vi "Get Mentions Old.vi"(8 "error in":errorcluster, 9 "Mentions to Read (10)":i32=10 min=0 max=200 step=1, 11 "Twitter Handle In":T2={"OAuth Credentials"={"Consumer Key"="", "Signature Method"=enum."HMAC-SHA1", "Token"="", "Version"="", "Token Secret"="", "Consumer Secret"=""}, "since ID"="", "max ID"="", "Screen Name"=""}) -> (0 "error out":errorcluster, 1 "Actual Num of Mentions Read":i32, 2 "Old Mentions Read":T1[](array[typedef]), 3 "Twitter Handle Out":T2={"OAuth Credentials"={"Consumer Key"="", "Signature Method"=enum."HMAC-SHA1", "Token"="", "Version"="", "Token Secret"="", "Consumer Secret"=""}, "since ID"="", "max ID"="", "Screen Name"=""}, 5 "Time Stamp of Oldest Mention":timestamp)   [LabVIEW 2011, in "i3-twitter.lvlib"]
doc: "Get authenticating user's old mentions."
uses:
  i3-twitter.lvlib
  Controls/Twitter Handle.ctl
  i3-oauth/Controls/OAuth Credentials.ctl
  i3-oauth/Controls/Signature Method.ctl
  Controls/Tweet.ctl
  i3-oauth/Controls/HTTP Method.ctl
  i3-oauth/i3-oauth.lvlib
  <vilib>/httpClient/LabVIEWHTTPClient.lvlib
  i3-json/i3-json.lvlib
panel:
  out "headers":string
  out "body":string
  out "Full URL":string
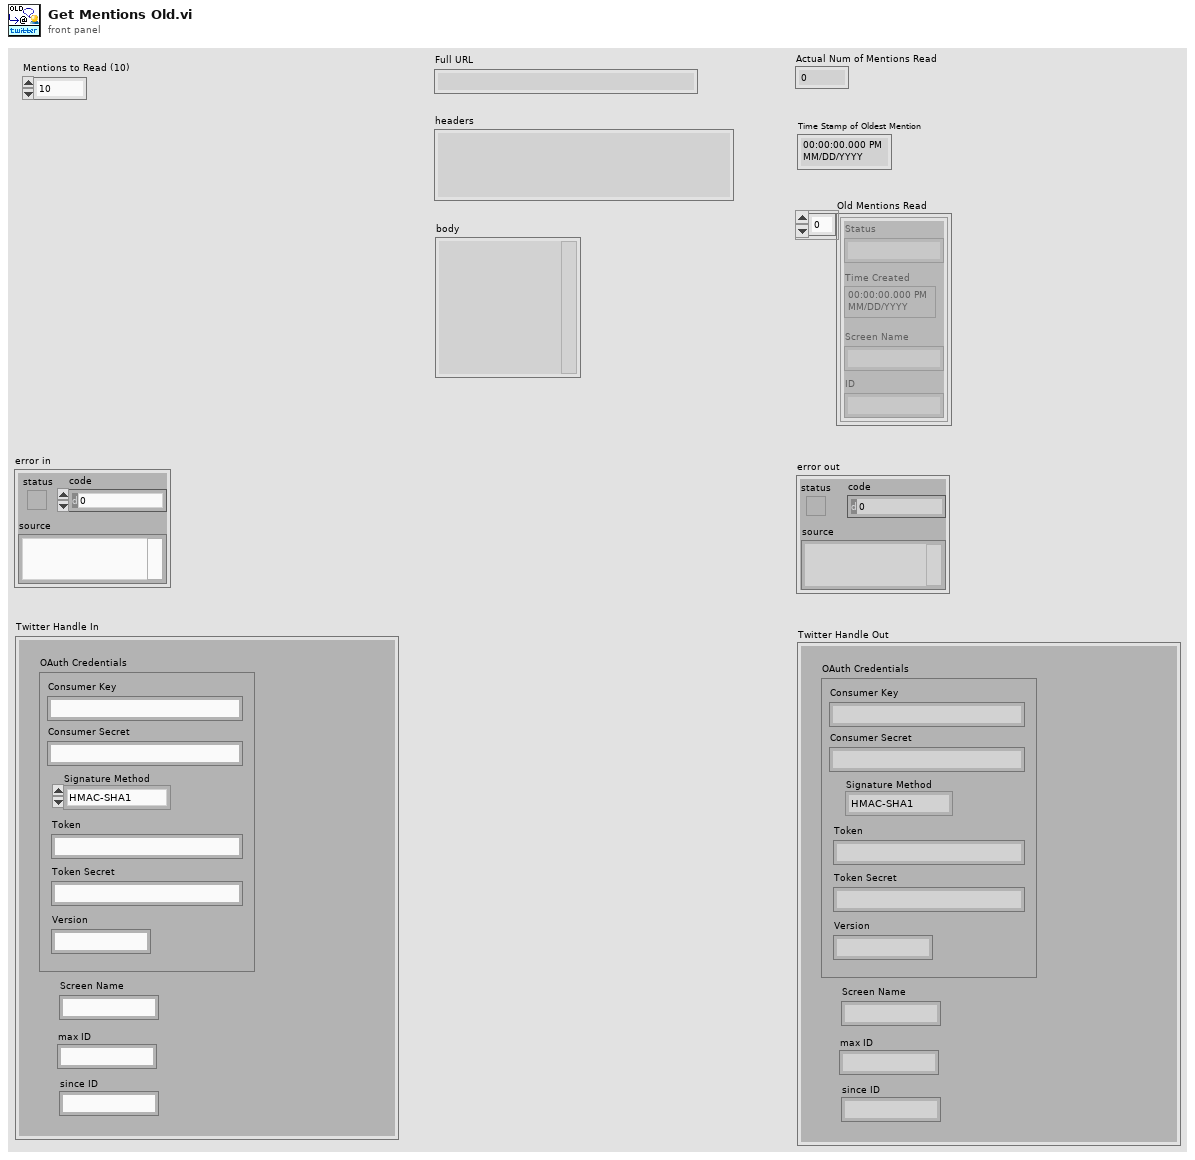
[diagram p1: front panel]
types:
  T1 = typedef "i3-twitter.lvlib/Tweet.ctl" = cluster{"Status":string, "Time Created":timestamp, "Screen Name":string, "ID":string}
  T2 = typedef "i3-twitter.lvlib/Twitter Handle.ctl" = cluster{"OAuth Credentials":T3, "since ID":string, "max ID":string, "Screen Name":string}
  T3 = typedef "i3-oauth.lvlib/OAuth Credentials.ctl" = cluster{"Consumer Key":string, "Signature Method":T4, "Token":string, "Version":string, "Token Secret":string, "Consumer Secret":string}
  T4 = typedef "i3-oauth.lvlib/Signature Method.ctl" = enum16{"HMAC-MD5", "HMAC-SHA1", "HMAC-SHA224", "HMAC-SHA256", "HMAC-SHA384", "HMAC-SHA512"}
  T5 = typedef "i3-oauth.lvlib/HTTP Method.ctl" = enum16{"GET", "POST", "PUT", "DELETE"}
  T6 = typedef "i3-oauth.lvlib/key-value-pairs.ctl" = cluster{"key":string, "value":string}
  T7 = typedef "LabVIEWHTTPClient.lvlib/ClientHandle.ctl" = refnum<k1>
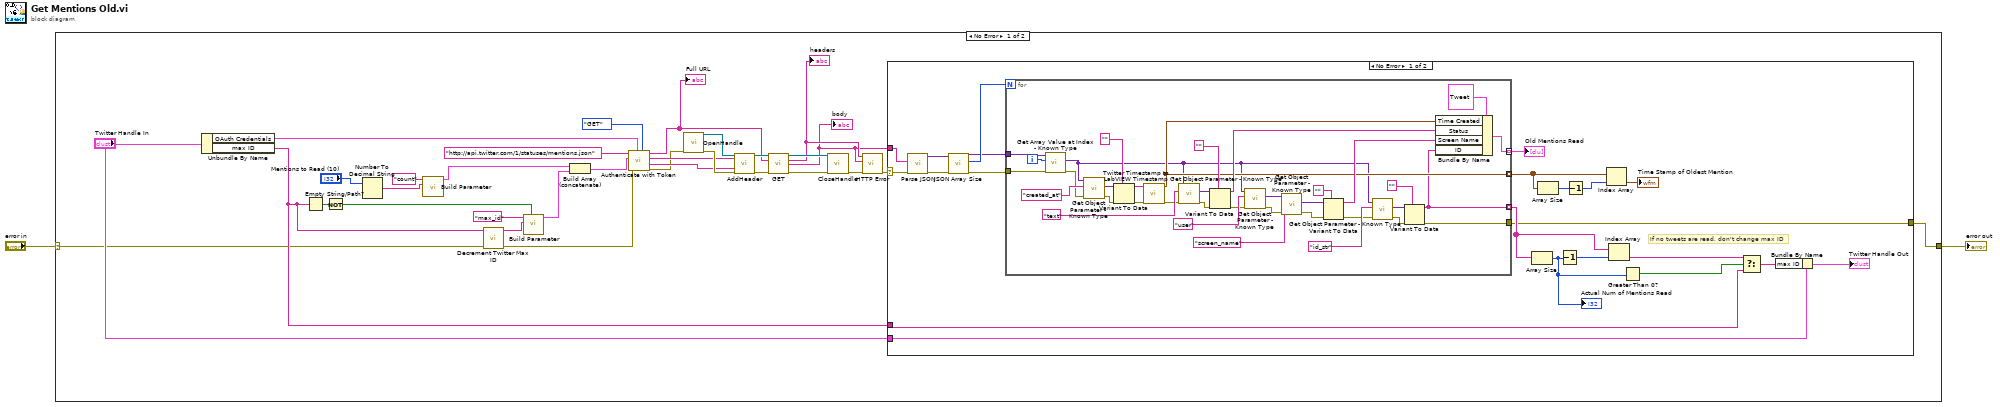
[diagram p0: block diagram]
diagram:
  n1 = case shown="No Error" "error in" {
    selector: "error in" -> [w3 w94]
    tunnel: [w4 w94] -> w2
    frame No Error {
      n2 = Unbundle By Name("Twitter Handle In") -> ("OAuth Credentials"=w8:T3, "max ID"=w6:string)
      n3 = Empty String/Path?(string/path=w6) -> (empty?=w18:bool)
      n4 = Not(x=w18) -> (.not. x?=w14:bool)
      n5 = Number To Decimal String(number="Mentions to Read (10)") -> (decimal integer string=w21:string)  [unwired: 1 in]
      n6 = call "Build Parameter.vi"("Value"=w21, "Key"="count") -> ("Parameter Array"=w7:T6[])  [unwired: 9 in]
      n7 = call "Decrement Twitter Max ID.vi"("error in (no error)"=w3, "ID In"=w6) -> ("error out"=w13:errorcluster, "ID Out"=w15:string)  [unwired: 8 in]
      n8 = call "Build Parameter.vi"("Return Parameter? (T)"=w14, "Value"=w15, "Key"="max_id") -> ("Parameter Array"=w17:T6[])  [unwired: 8 in]
      n9 = Build Array (concatenate)(w7, w17) -> (w20:T6[])
      n10 = call "Authenticate with Token.vi"("HTTP Method"=HTTP_Method."GET", "OAuth Credentials"=w8, "error in (no error)"=w13, "URL Parameters"=w20, "Base URL"="http://api.twitter.com/1/statuses/mentions.json") -> ("error out"=w19:errorcluster, "Header Value"=w26:string, "Header Parameter"=w27:string, "Full URL"=w24:string)  [unwired: 2 in, 1 out]
      "Full URL" <- w24
      n11 = call <vilib>:"OpenHandle.vi"("error in (no error)"=w19) -> ("client handle out"=w33:T7, "error out"=w32:errorcluster)  [unwired: 13 in]
      n12 = call <vilib>:"AddHeader.vi"("client handle"=w33, "header"=w27, "value"=w26, "error in (no error)"=w32) -> ("client handle out"=w31:T7, "error out"=w30:errorcluster)  [unwired: 10 in]
      n13 = call <vilib>:"GET.vi"("client handle"=w31, "url"=w24, "error in (no error)"=w30) -> ("client handle out"=w29:T7, "headers"=w12:string, "body"=w9:string, "error out"=w28:errorcluster)  [unwired: 9 in]
      "body" <- w9
      "headers" <- w12
      n14 = call <vilib>:"CloseHandle.vi"("client handle"=w29, "error in (no error)"=w28) -> ("error out"=w11:errorcluster)  [unwired: 13 in]
      n15 = call "HTTP Error.vi"("error in (no error)"=w11, "Body"=w9, "Header"=w12) -> ("error out"=w10:errorcluster)  [unwired: 6 in, 2 out]
      n16 = case shown="No Error" w10 {
        selector: w10 -> [w42 w93]
        tunnel: w6 -> [w45 _]
        tunnel: "Twitter Handle In" -> [w44 _]
        tunnel: [w39 w93] -> w4
        tunnel: w9 -> [w41 _]
        frame No Error {
          # "If no tweets are read, don't change max ID"
          n17 = call "Parse JSON.vi"("error in (no error)"=w42, "JSON String"=w41) -> ("error out"=w53:errorcluster, "JSON Tree"=w55:variant)  [unwired: 6 in, 2 out]
          n18 = call "JSON Array Size.vi"("error in (no error)"=w53, "JSON Tree In (JSON Array)"=w55) -> ("error out"=w52:errorcluster, "Array Size"=w56:i32, "JSON Tree Passthrough (JSON Array)"=w46:variant)  [unwired: 7 in]
          n19 = for {
            N: w56 -> [_]
            tunnel: [w59] -> w54 mode=indexing
            tunnel: w52 -> [w62]
            tunnel: [w72] -> w51 mode=indexing
            tunnel: [w71] -> w39
            tunnel: w46 -> [w61]
            tunnel: [w60] -> w37 mode=indexing
            i -> [w81]
            n20 = call "Get Array Value at Index - Known Type.vi"("error in (no error)"=w62, "Index"=w81, "JSON Tree In (JSON Array)"=w61) -> ("error out"=w75:errorcluster, "Value"=w58:variant)  [unwired: 3 in, 4 out]
            n21 = call "Get Object Parameter - Known Type.vi"("error in (no error)"=w75, "Parameter Name"="created_at", "JSON Tree In (JSON Object)"=w58) -> ("error out"=w70:errorcluster, "Value"=w68:variant)  [unwired: 3 in, 4 out]
            n22 = Variant To Data(error in=w70, type="", Variant=w68) -> (data=w80:string, error out=w66:errorcluster)
            n23 = call "Twitter Timestamp to LabVIEW Timestamp.vi"("error in"=w66, "Twitter Time Stamp"=w80) -> ("error out"=w65:errorcluster, "LabVIEW Time Stamp"=w60:timestamp)  [unwired: 6 in]
            n24 = call "Get Object Parameter - Known Type.vi"("error in (no error)"=w65, "Parameter Name"="text", "JSON Tree In (JSON Object)"=w58) -> ("error out"=w69:errorcluster, "Value"=w90:variant)  [unwired: 3 in, 4 out]
            n25 = Variant To Data(error in=w69, type="", Variant=w90) -> (data=w63:string, error out=w67:errorcluster)
            n26 = call "Get Object Parameter - Known Type.vi"("error in (no error)"=w67, "Parameter Name"="user", "JSON Tree In (JSON Object)"=w58) -> ("error out"=w74:errorcluster, "Value"=w57:variant)  [unwired: 3 in, 4 out]
            n27 = call "Get Object Parameter - Known Type.vi"("error in (no error)"=w74, "Parameter Name"="screen_name", "JSON Tree In (JSON Object)"=w57) -> ("error out"=w73:errorcluster, "Value"=w85:variant)  [unwired: 3 in, 4 out]
            n28 = Variant To Data(error in=w73, type="", Variant=w85) -> (data=w86:string, error out=w64:errorcluster)
            n29 = call "Get Object Parameter - Known Type.vi"("error in (no error)"=w64, "Parameter Name"="id_str", "JSON Tree In (JSON Object)"=w58) -> ("error out"=w78:errorcluster, "Value"=w77:variant)  [unwired: 3 in, 4 out]
            n30 = Variant To Data(error in=w78, type="", Variant=w77) -> (data=w59:string, error out=w71:errorcluster)
            n31 = Bundle By Name(cluster=T1 {"Status"="", "Time Created"=timestamp(0 s since 1904-01-01), "Screen Name"="", "ID"=""}, "Time Created"=w60, "Status"=w63, "Screen Name"=w86, "ID"=w59) -> (w72:T1)
          }
          "Old Mentions Read" <- w51
          n32 = Array Size(array=w54) -> (size(s)=w49:i32)
          "Actual Num of Mentions Read" <- w49
          n33 = Array Size(array=w37) -> (size(s)=w36:i32)
          n34 = Decrement(x=w49) -> (x-1=w38:i32)
          n35 = Decrement(x=w36) -> (x-1=w35:i32)
          n36 = Index Array(array=w37, index=w35) -> (element=→"Time Stamp of Oldest Mention":timestamp)
          n37 = Index Array(array=w54, index=w38) -> (element=w48:string)
          n38 = Greater Than 0?(x=w49) -> (x > 0?=w50:bool)
          n39 = Select(t=w48, s=w50, f=w45) -> (s? t:f=w47:string)
          n40 = Bundle By Name(cluster=w44, "max ID"=w47) -> (→"Twitter Handle Out":T2)
        }
        frame Error {
        }
      }
    }
    frame Error {
    }
  }
  "error out" <- w2
